vi "Test DUT Self Test Fails if Not Powered.vi"(8 "error in (no error)":errorcluster, 11 "Device Under Test Test In":refnum<class "Device Under Test Test.lvclass">) -> (0 "error out":errorcluster, 3 "Device Under Test Test Out":refnum<class "Device Under Test Test.lvclass">)   [LabVIEW 2020, in "Device Under Test Test.lvclass"]
uses:
  Device Under Test Test.lvclass
  C:/Program Files (x86)/National Instruments/LabVIEW 2020/vi.lib/Astemes/LUnit/Test Case.lvclass
  Device Under Test/Device Under Test.lvclass
  C:/Program Files (x86)/National Instruments/LabVIEW 2020/vi.lib/Astemes/Triarc Framework/Process/Process.lvclass
  <vilib>/Astemes/LUnit/Test Case.lvclass/Test Case.ctl
  <vilib>/Astemes/Triarc Framework/Process/Process.lvclass/Process.ctl
  <vilib>/Astemes/LUnit/Core/LUnit Test Case/Private/Append Pass Result.vi
  <vilib>/Astemes/LUnit/Core/LUnit Test Case/Private/Append Fail Result.vi
  <vilib>/Astemes/Triarc Framework/Process/Private/SubVIs/Wait for finish.vi
  <vilib>/Astemes/Triarc Framework/Process/Private/SubVIs/Set Lifecycle State.vi
  <vilib>/Astemes/Triarc Framework/Process/Protected/Messaging/Send Message.vi
  <vilib>/Astemes/LUnit/Core/LUnit Test Case/Private/Run In UI.vi
  <vilib>/Astemes/Triarc Framework/Process/Private/SubVIs/Handle Debug Data.vi
  <vilib>/Utility/error.llb/Clear Errors.vi
  <vilib>/Astemes/Triarc Framework/Process/Public/Lifecycle/Get Lifecycle State.vi
  <vilib>/Utility/error.llb/Error Cluster From Error Code.vi
  <vilib>/Astemes/Triarc Framework/Callback/Callback.lvclass
  <vilib>/Astemes/Triarc Framework/Process/Process.lvclass
  <vilib>/Astemes/LUnit/Test Case.lvclass
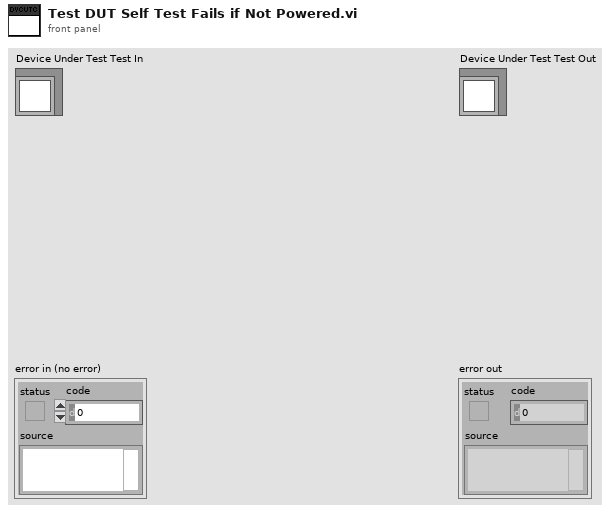
[diagram p1: front panel]
types:
  T1 = typedef "Device Under Test.lvclass/Self Test Reply Payload.ctl" = cluster{"Result":bool, "Self Test Error":errorcluster}
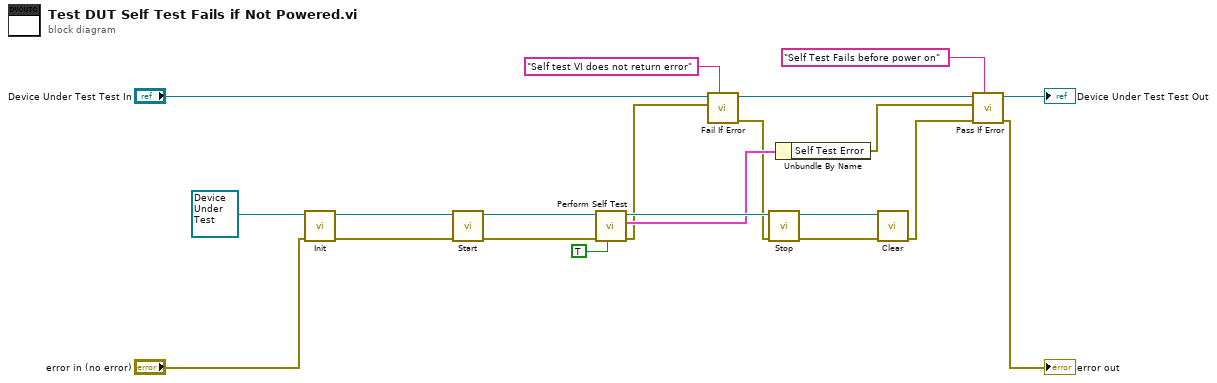
[diagram p0: block diagram]
diagram:
  n1 = call-dynamic "Init.vi"("error in (no error)"="error in (no error)", "View In"=refnum<class "Device Under Test.lvclass"> refnum ("Device Under Test.lvclass")) -> ("error out"=w14:errorcluster, "View Out"=w15:refnum<class "Device Under Test.lvclass">)  [unwired: 8 in]
  n2 = call <vilib>:"Start.vi"("error in (no error)"=w14, "Process In"=w15) -> ("error out"=w20:errorcluster, "Process Out"=w7:refnum<class "Device Under Test.lvclass">)  [unwired: 7 in, 1 out]
  n3 = call "Perform Self Test.vi"("Wait for Reply?"=TRUE, "error in (no error)"=w20, "Device Under Test In"=w7) -> ("error out"=w3:errorcluster, "data"=w6:T1, "Device Under Test Out"=w19:refnum<class "Device Under Test.lvclass">)  [unwired: 5 in, 1 out]
  n4 = call <vilib>:"Fail If Error.vi"("Description"="Self test VI does not return error", "Assert error"=w3, "LUnit Test Case In"="Device Under Test Test In") -> ("error out"=w2:errorcluster, "LUnit Test Case Out"=w4:refnum<class "Device Under Test Test.lvclass">)  [unwired: 7 in]
  n5 = call <vilib>:"Stop.vi"("error in (no error)"=w2, "Process In"=w19) -> ("error out"=w17:errorcluster, "Process Out"=w18:refnum<class "Device Under Test.lvclass">)  [unwired: 7 in, 1 out]
  n6 = Unbundle By Name(w6) -> ("Self Test Error"=w5:errorcluster)
  n7 = call-dynamic "Clear.vi"("error in (no error)"=w17, "View In"=w18) -> ("error out"=w12:errorcluster)  [unwired: 9 in]
  n8 = call <vilib>:"Pass If Error.vi"("Description"="Self Test Fails before power on", "error in (no error)"=w12, "Assert error"=w5, "LUnit Test Case In"=w4) -> ("error out"=→"error out":errorcluster, "LUnit Test Case Out"=→"Device Under Test Test Out":refnum<class "Device Under Test Test.lvclass">)  [unwired: 6 in]
